vi "DigitizerMemory.vi"(3 "Digitizer Settings":T1={"Digitizer delay (us) "=0.0, "rf points per line"=2048, "lines per plane"=128, "Samp Rate (Hz)"=100000000.0, "Additional dig delay (us)"=0.0, "Voltage Scale"=0.4, "Pre-Looks"=0, "Offset delay (us)"=0.0, "bits A/D"=8, "Avg Num"=1, "DigTimeOut"=5.0, "Rel Dig Delay"=0.0, "Dig Ch"=0, "LeCroyCluster"={"LeCroy Channels"=[TRUE, FALSE, FALSE, FALSE], "LC read pt offset"=0.0, "Sweep Avg"=FALSE}, "Main Digitizer"=enum."NI Digitizer", "Dig Config"=enum."Single channel", "Digitizer ID Cluster"={"Acqiris/Alazar/SP ID"=[], "NI Instr Handles"=[], "LeCroy VISA"="", "GaGe Handle"={"Handle"=0, "Sample size"=0, "Resolution"=0, "Offset"=0, "Channels"=0, "Boards"=0}, "ATS Ref"="ATS9350", "Acqiris Address"=["PCI::INSTR0"], "ADQRef"=refnum, "adq_cu_ptr"=refnum}, "Trigger Settings"={"Trig Source"=1, "Trig Coupling"=0, "Trig Slope"=0, "Level (mV)"=1500.0}, "Bulk Acq"=FALSE, "Bulk Start Indexes"=[], "Data Ref RF"=refnum, "NI ID/Channel"=[], "Total Dig CH"=1, "Xtra Ann Trig delay (us)"=10.0, "Fix Z Delay?"=FALSE, "One Way Transmission?"=FALSE, "Data Ref Log"=refnum} {"Trigger Settings"."Trig Slope" items=["Positive", "Negative"]; "Trigger Settings"."Level (mV)" format="%.2f"; "Trigger Settings"."Trig Coupling" items=["DC 1 MOhm", "AC 1 MOhm", "DC 50 Ohm", "AC 50 Ohm"]; "Trigger Settings"."Trig Source" items=["Chan 1", "External"]; "Rel Dig Delay" format="%.2f"; "DigTimeOut" format="%.2f"; "Avg Num" min=1; "Offset delay (us)" format="%.2f"; "Additional dig delay (us)" format="%.2f"; "Digitizer delay (us)" format="%.2f"}) -> (1 "Memory":i32)   [LabVIEW 2022 SP3]
uses:
  DigitizerSettings.ctl
  Digitizer.ctl
  DigConfig.ctl
  DigitizerID.ctl
  C:/Windows/System32/ADQAPI_dotNet_helper.dll
  <instrlib>/Acqiris Bx/Acqiris Bx.lvlib
  <instrlib>/LeCroy Wave Series/LeCroy Wave Series.lvlib
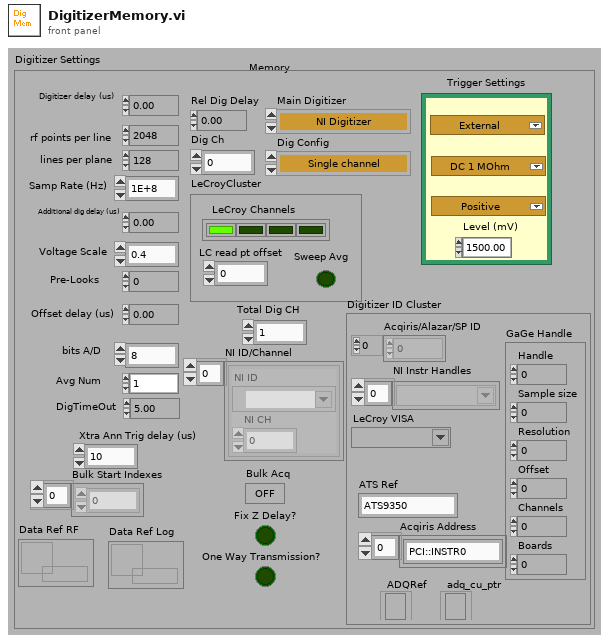
[diagram p1: front panel]
types:
  T1 = typedef "DigitizerSettings.ctl" = cluster{"Digitizer delay (us) ":dbl, "rf points per line":i32, "lines per plane":i32, "Samp Rate (Hz)":dbl, "Additional dig delay (us)":dbl, "Voltage Scale":dbl, "Pre-Looks":i32, "Offset delay (us)":dbl, "bits A/D":i8, "Avg Num":i32, "DigTimeOut":sgl, "Rel Dig Delay":sgl, "Dig Ch":i32, "LeCroyCluster":cluster{"LeCroy Channels":bool[], "LC read pt offset":dbl, "Sweep Avg":bool}, "Main Digitizer":T2, "Dig Config":T3, "Digitizer ID Cluster":T4, "Trigger Settings":cluster{"Trig Source":u16, "Trig Coupling":u16, "Trig Slope":u16, "Level (mV)":dbl}, "Bulk Acq":bool, "Bulk Start Indexes":i32[], "Data Ref RF":refnum<data-value>, "NI ID/Channel":cluster{"NI ID":refnum<k15>, "NI CH":i32}[], "Total Dig CH":i32, "Xtra Ann Trig delay (us)":dbl, "Fix Z Delay?":bool, "One Way Transmission?":bool, "Data Ref Log":refnum<data-value>}
  T2 = typedef "Digitizer.ctl" = enum16{"Acqiris Digitizer", "NI Digitizer", "LeCroy", "GaGe", "AlazarTech", "No Digitizer", "Teledyne"}
  T3 = typedef "DigConfig.ctl" = enum16{"Single channel", "2 Chans w/ 2 Acqiris", "2 Chans w/ 1 Acqiris", "5-CH Pulser New", "5-CH pulser w/ ann array", "5-pass style ann array", "Empty"}
  T4 = typedef "DigitizerID.ctl" = cluster{"Acqiris/Alazar/SP ID":u32[], "NI Instr Handles":refnum<k15>[], "LeCroy VISA":refnum<visa-resource-name>, "GaGe Handle":cluster{"Handle":u32, "Sample size":u32, "Resolution":i32, "Offset":i32, "Channels":u32, "Boards":u32}, "ATS Ref":string, "Acqiris Address":string[], "ADQRef":refnum<k24>, "adq_cu_ptr":refnum<k24>}
  T5 = cluster{"Handle":u32, "Sample size":u32, "Resolution":i32, "Offset":i32, "Channels":u32, "Boards":u32}
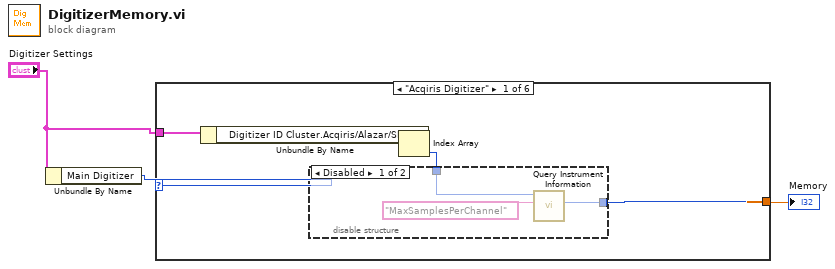
[diagram p0: block diagram]
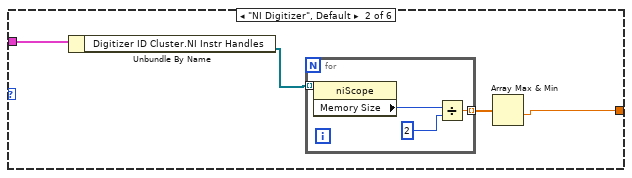
[diagram p3: hidden frame]
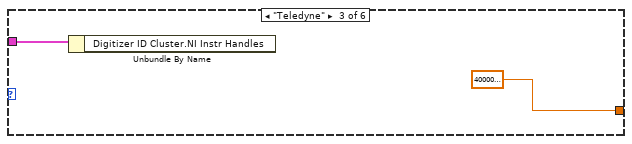
[diagram p4: hidden frame]
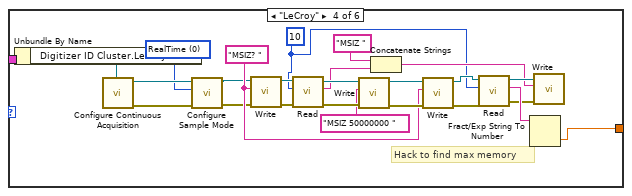
[diagram p5: hidden frame]
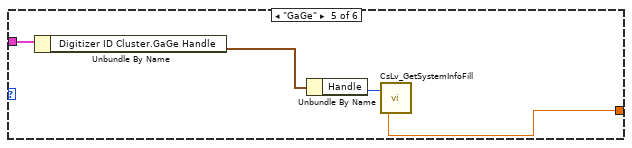
[diagram p6: hidden frame]
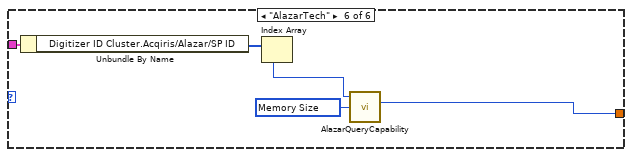
[diagram p7: hidden frame]
diagram:
  n1 = Unbundle By Name("Digitizer Settings") -> ("Main Digitizer"=w1:T2)
  n2 = case shown="\"Acqiris Digitizer\"" w1 {
    tunnel: [w7 w13 4000000000.0 w29 w49 w50] -> w3
    tunnel: "Digitizer Settings" -> [w5 w12 w20 w22 w47 w54]
    frame "Acqiris Digitizer" {
      n3 = Unbundle By Name(w5) -> ("Digitizer ID Cluster.Acqiris/Alazar/SP ID"=w6:u32[])
      n4 = Index Array(array=w6) -> (element=w4:u32)  [unwired: 1 in]
      n5 = disable-structure shown="Disabled" {
        disable-tunnel: [w9 _] -> w7
        disable-tunnel: w4 -> [w8 _]
        frame Disabled {
          n6 = call <instrlib>:"Query Instrument Information.vi"("Instrument ID"=w8, "Parameter String"="MaxSamplesPerChannel") -> ("Info Value (I32)"=w9:i32)  [unwired: 2 in, 5 out]
        }
        frame Enabled {
        }
      }
    }
    frame "NI Digitizer", Default {
      n7 = Unbundle By Name(w12) -> ("Digitizer ID Cluster.NI Instr Handles"=w11:refnum<k15>[])
      n8 = for {
        tunnel: [w16] -> w14 mode=indexing
        tunnel: w11 -> [w15] mode=indexing
        n9 = property class="niScope"(reference=w15) -> ("Memory Size"=w18:i32)  [unwired: 1 in, 2 out]
        n10 = Divide(x=w18, y=2) -> (x/y=w16:dbl)
      }
      n11 = Array Max & Min(array=w14) -> (min value=w13:dbl)  [unwired: 3 out]
    }
    frame "Teledyne" {
      n12 = Unbundle By Name(w20) -> ()  [unwired: 1 out]
    }
    frame "LeCroy" {
      w25 = u16 0 items=["RealTime", "RIS", "Sequence", "Roll", "WaveStream"] ("Sample Mode (0: RealTime)")
      w28 = 10
      w38 = "MSIZ? " ("Write Buffer")
      # "Hack to find max memory"
      n13 = Unbundle By Name(w22) -> ("Digitizer ID Cluster.LeCroy VISA"=w21:refnum<visa-resource-name>)
      n14 = call <instrlib>:"Configure Continuous Acquisition.vi"("VISA resource name"=w21) -> ("error out"=w27:errorcluster, "VISA resource name out"=w26:refnum<visa-resource-name>)  [unwired: 9 in]
      n15 = call <instrlib>:"Configure Sample Mode.vi"("error in (no error)"=w27, "Sample Mode (0: RealTime)"=w25, "VISA resource name"=w26) -> ("error out"=w23:errorcluster, "VISA resource name out"=w24:refnum<visa-resource-name>)  [unwired: 7 in]
      n16 = call <instrlib>:"Write.vi"("error in (no error)"=w23, "Write Buffer"=w38, "VISA resource name"=w24) -> ("error out"=w45:errorcluster, "VISA resource name out"=w44:refnum<visa-resource-name>)  [unwired: 6 in, 1 out]
      n17 = call <instrlib>:"Read.vi"("error in (no error)"=w45, "Byte Count"=w28, "VISA resource name"=w44) -> ("error out"=w42:errorcluster, "Read Buffer"=w31:string, "VISA resource name out"=w43:refnum<visa-resource-name>)  [unwired: 5 in, 1 out]
      n18 = call <instrlib>:"Write.vi"("error in (no error)"=w42, "Write Buffer"="MSIZ 50000000 ", "VISA resource name"=w43) -> ("error out"=w39:errorcluster, "VISA resource name out"=w40:refnum<visa-resource-name>)  [unwired: 6 in, 1 out]
      n19 = Concatenate Strings("MSIZ ", w31) -> (w30:string)
      n20 = call <instrlib>:"Write.vi"("error in (no error)"=w39, "Write Buffer"=w38, "VISA resource name"=w40) -> ("error out"=w36:errorcluster, "VISA resource name out"=w37:refnum<visa-resource-name>)  [unwired: 6 in, 1 out]
      n21 = call <instrlib>:"Read.vi"("error in (no error)"=w36, "Byte Count"=w28, "VISA resource name"=w37) -> ("error out"=w33:errorcluster, "Read Buffer"=w35:string, "VISA resource name out"=w34:refnum<visa-resource-name>)  [unwired: 5 in, 1 out]
      n22 = Fract/Exp String To Number(string=w35) -> (number=w29:dbl)  [unwired: 3 in, 1 out]
      n23 = call <instrlib>:"Write.vi"("error in (no error)"=w33, "Write Buffer"=w30, "VISA resource name"=w34) -> ()  [unwired: 6 in, 3 out]
    }
    frame "GaGe" {
      n24 = Unbundle By Name(w47) -> ("Digitizer ID Cluster.GaGe Handle"=w46:T5)
      n25 = Unbundle By Name(w46) -> ("Handle"=w48:u32)
      n26 = call "CsLv_GetSystemInfoFill.vi"("Handle"=w48) -> ("Memory Size"=w49:dbl)  [unwired: 6 out]
    }
    frame "AlazarTech" {
      w52 = u32 268435498 items=["Get Serial Number"=268435492, "Get Latest Cal. Date"=268435494, "Get Latest Cal. Month"=268435501, "Get Latest Cal. Day"=268435502, "Get Latest Cal. Year"=268435503, "Memory Size"=268435498, "Board Type"=268435499, "ASOPC Type"=268435500, "Get PCIe Link Speed "=268435504, "Get PCIe Link Width"=268435505, "Get Max Pretrigger Samples"=268435526, "Get CPF Device"=268435569] ("Capability")
      n27 = Unbundle By Name(w54) -> ("Digitizer ID Cluster.Acqiris/Alazar/SP ID"=w53:u32[])
      n28 = Index Array(array=w53) -> (element=w51:u32)  [unwired: 1 in]
      n29 = call "AlazarQueryCapability.vi"("Handle"=w51, "Capability"=w52) -> ("Value"=w50:u32)  [unwired: 1 in, 3 out]
    }
  }
  "Memory" <- w3
